vi "RequestNodeUpdate.vi"(0 "OccupancyGridWorldMap in":refnum<class "NI_Robotics_OccupancyGridWorldMap.lvclass">, 5 "x":i32, 7 "y":i32, 9 "Cost":dbl, 11 "error in (no error)":errorcluster) -> (4 "OccupancyGridWorldMap out":refnum<class "NI_Robotics_OccupancyGridWorldMap.lvclass">, 15 "error out":errorcluster)   [LabVIEW 2017, in "NI_Robotics_OccupancyGridWorldMap.lvclass"]
uses:
  <vilib>/robotics/Navigation/shared/WorldMap/OccupancyGridWorldMap/NI_Robotics_OccupancyGridWorldMap.lvclass
  <vilib>/robotics/Navigation/shared/WorldMap/OccupancyGridWorldMap/NI_Robotics_OccupancyGridWorldMap.lvclass/NI_Robotics_OccupancyGridWorldMap.ctl
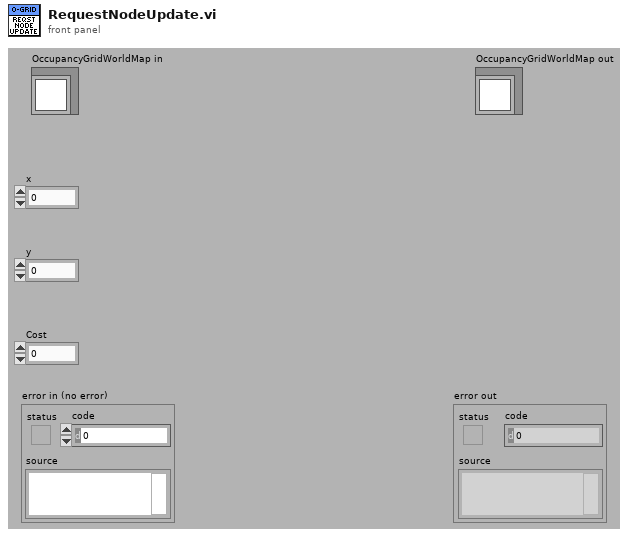
[diagram p1: front panel]
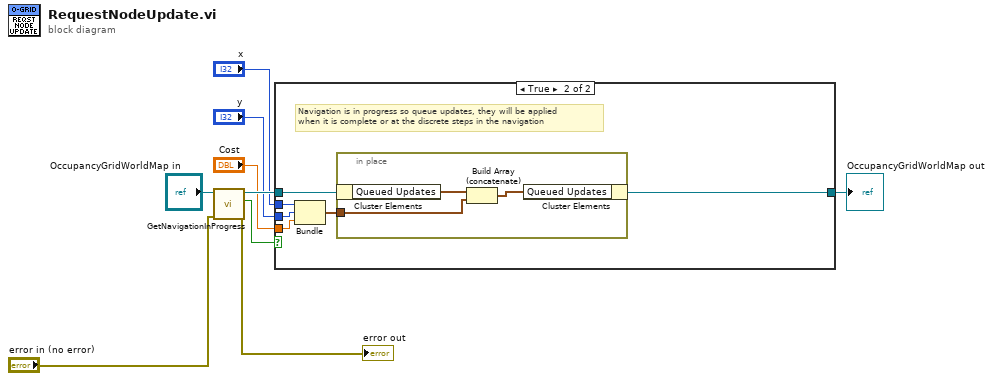
[diagram p0: block diagram]
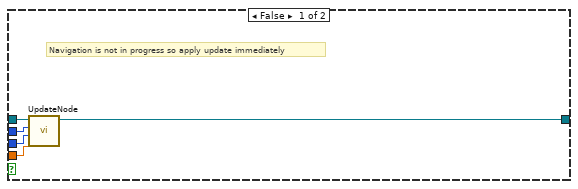
[diagram p2: hidden frame]
diagram:
  n1 = call-dynamic "GetNavigationInProgress.vi"("error in (no error)"="error in (no error)", "AbstractWorldMap in"="OccupancyGridWorldMap in") -> ("error out"=→"error out":errorcluster, "Navigation in Progress"=w9:bool, "AbstractWorldMap out"=w8:refnum<class "NI_Robotics_OccupancyGridWorldMap.lvclass">)  [unwired: 7 in]
  n2 = case shown="True" w9 {
    tunnel: w8 -> [w14 w17]
    tunnel: "x" -> [w12 w20]
    tunnel: "y" -> [w11 w19]
    tunnel: "Cost" -> [w10 w18]
    tunnel: [w13 w15] -> w3
    frame False {
      # "Navigation is not in progress so apply update immediately"
      n3 = call-dynamic "UpdateNode.vi"("Cost"=w10, "y"=w11, "x"=w12, "OccupancyGridWorldMap in"=w14) -> ("OccupancyGridWorldMap out"=w13:refnum<class "NI_Robotics_OccupancyGridWorldMap.lvclass">)  [unwired: 7 in]
    }
    frame True {
      # "Navigation is in progress so queue updates, they will be applied\nwhen it is complete or at the discrete steps in the navigation"
      n4 = Bundle("x"=w20, "y"=w19, "Cost"=w18) -> (w16:cluster{"x":i32, "y":i32, "Cost":dbl})  [unwired: 1 in]
      n5 = in-place {
        in-place-border: w16 -> [w21]
        n6 = in-place-cluster #1(w17) -> ("Queued Updates"=w23:cluster{"x":i32, "y":i32, "Cost":dbl}[])
        n7 = Build Array (concatenate)(w23, w21) -> (w22:cluster{"x":i32, "y":i32, "Cost":dbl}[])
        n8 = in-place-cluster #1("Queued Updates"=w22) -> (w15:refnum<class "NI_Robotics_OccupancyGridWorldMap.lvclass">)
      }
    }
  }
  "OccupancyGridWorldMap out" <- w3
